vi "Plot_XY_data.vi"(0 "Channel Values":string[][](array[string]), 1 "Ordinate Strings":string[](array[string]), 2 "Swap color and symbol":i32, 3 "Error Bar Chs":i32[](array[numeric])=[11], 5 "Accept Array":bool[][](array[boolean]), 7 "Filter 1 Strings":string[](array[string]), 9 "Filter 2 Strings":string[](array[string]), 11 "Ordinate":i32[](array[numeric])=[11], 12 "Absisca":u16, 13 "Transpose":bool) -> (15 "Accept Array Out":bool[][](array[boolean]))   [LabVIEW 2010]
uses:
  Results_plotter_Global.vi
panel:
  out "Colour Array":u32[][](array[colorbox])=[[26112, 39168, 52224, 65280, 65433], [153, 13311, 26367, 52479, 65535], [16711680, 16724838, 16737894, 16737945, 16751103], [16776960, 16777062, 16777113, 16777164, 16777215], [65280, 65280, 65280, 65280, 65280], [65280, 65280, 65280, 65280, 102]]
  out "Point Choice":u8[](array[numeric])=[1, 5, 13, 2, 6, 11, 15, 14]
  in  "Index Filter2":i32
  in  "Index Filter1":i32
  in  "Index Ordinate":i32
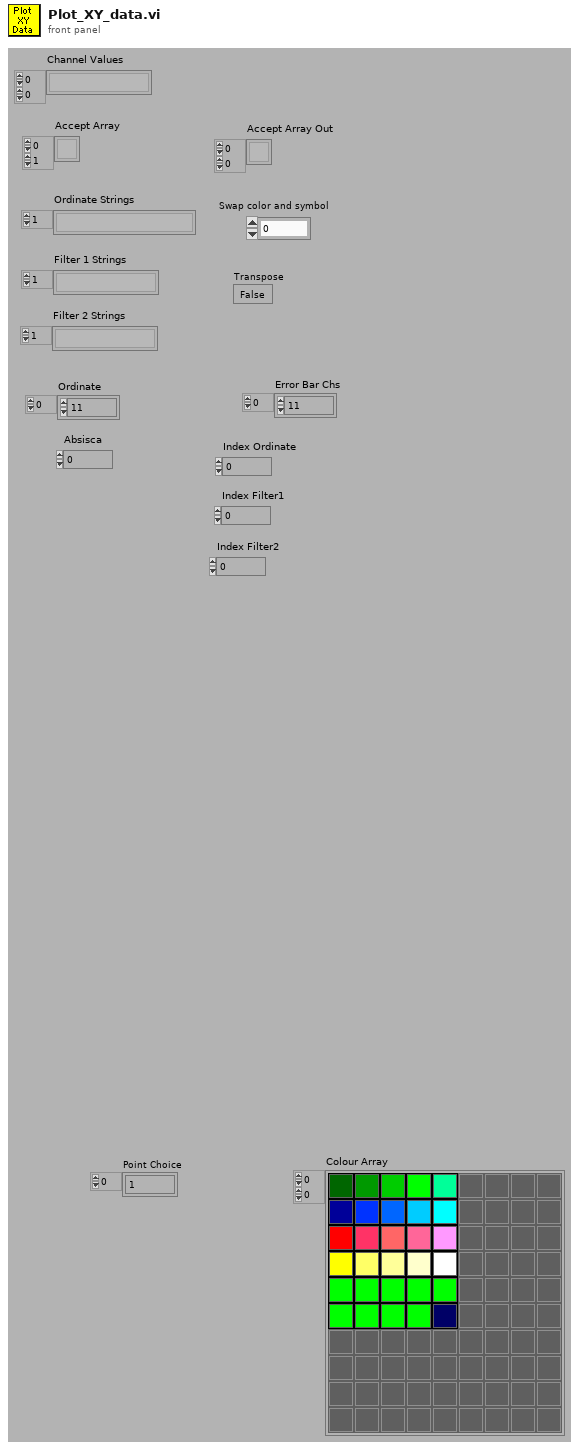
[diagram p1: front panel]
types:
  T1 = cluster{"Plot Color":u32, "Plot Interpolation":u8, "Point Style":u8, "Line Style":u8, "Fill/Pt. Color":u32, "Line Width":u8, "Bar Plot Style":u8, "Fill To":i16}
  T2 = cluster{"sorted array":dbl[], "sorted array":dbl[]}[]
  T3 = cluster{"Plot Color":u32, "Plot Interpolation":u8, "Point Style":u8, "Line Style":u8, "Fill/Pt. Color":u32, "Line Width":u8, "Bar Plot Style":u8, "Fill To":i16}[]
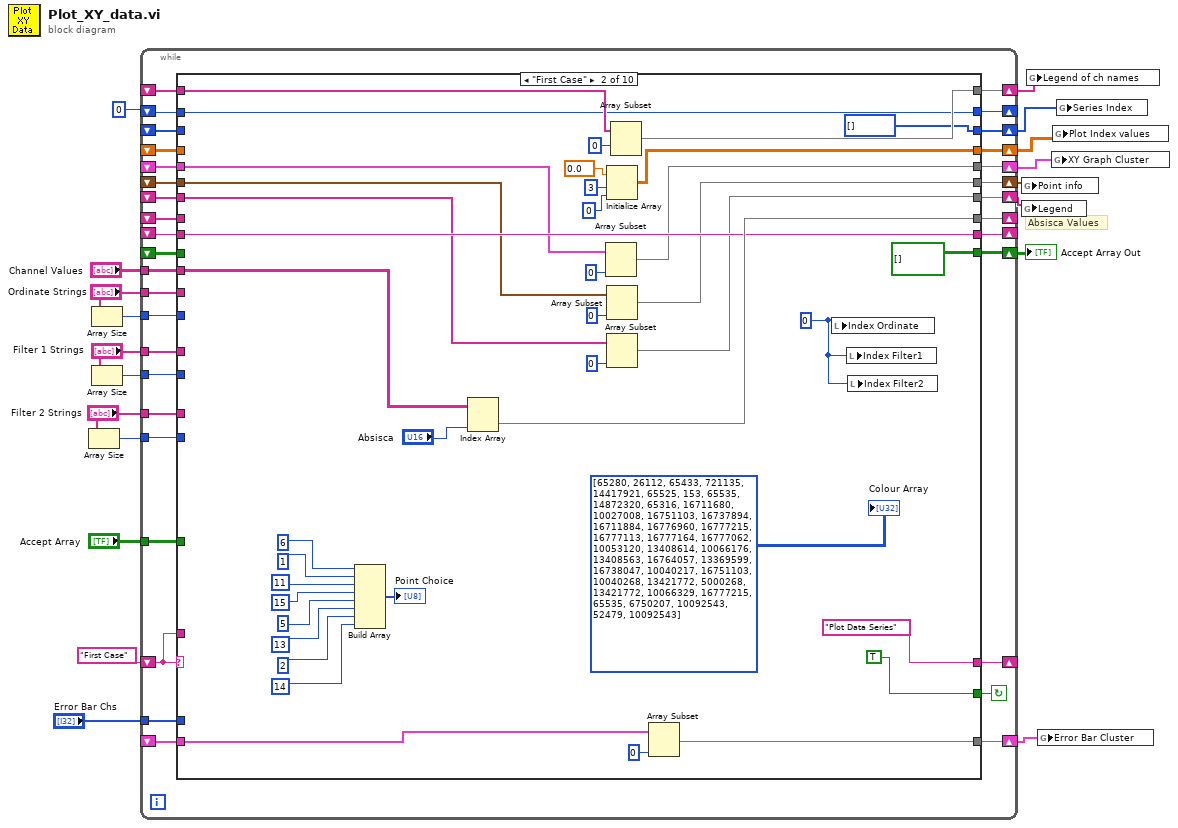
[diagram p0: block diagram]
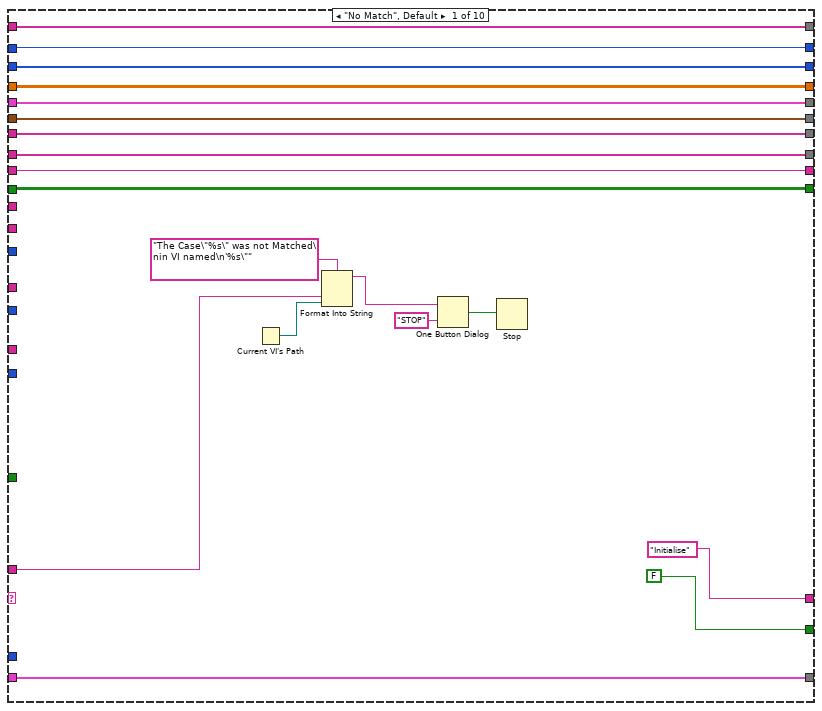
[diagram p2: hidden frame]
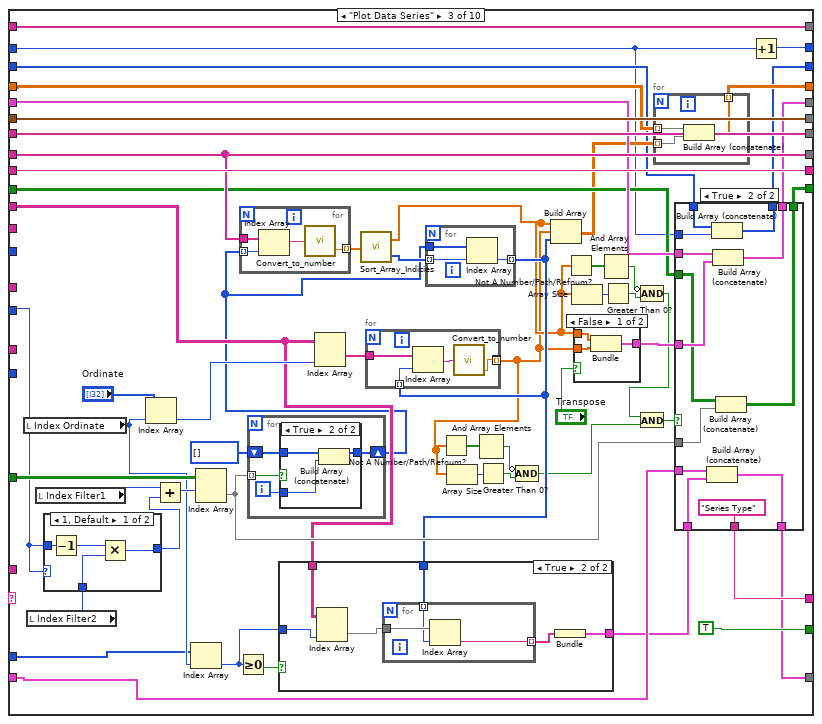
[diagram p3: hidden frame]
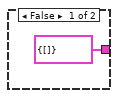
[diagram p4: hidden frame]
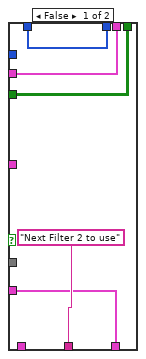
[diagram p6: hidden frame]
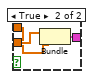
[diagram p7: hidden frame]
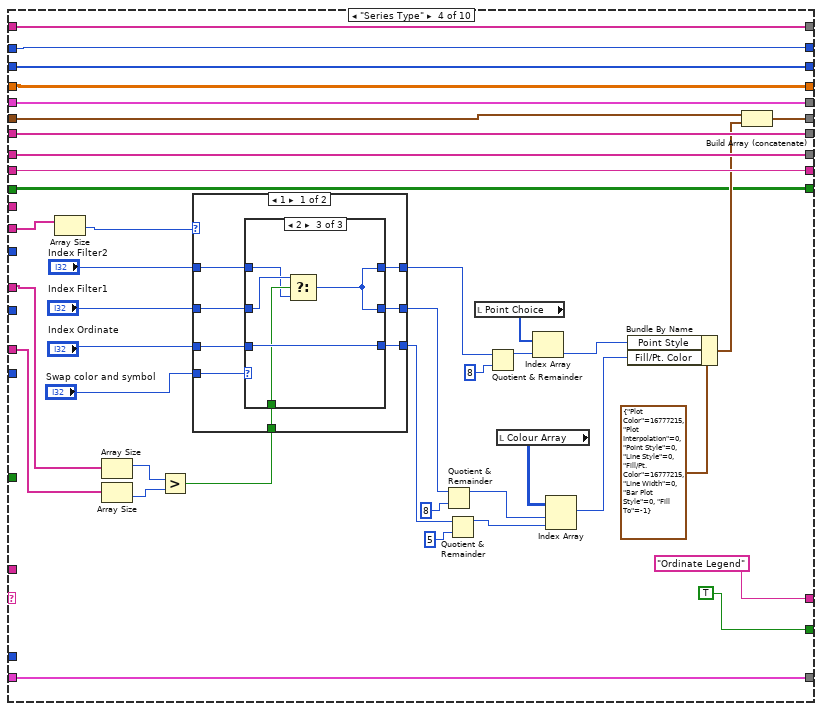
[diagram p9: hidden frame]
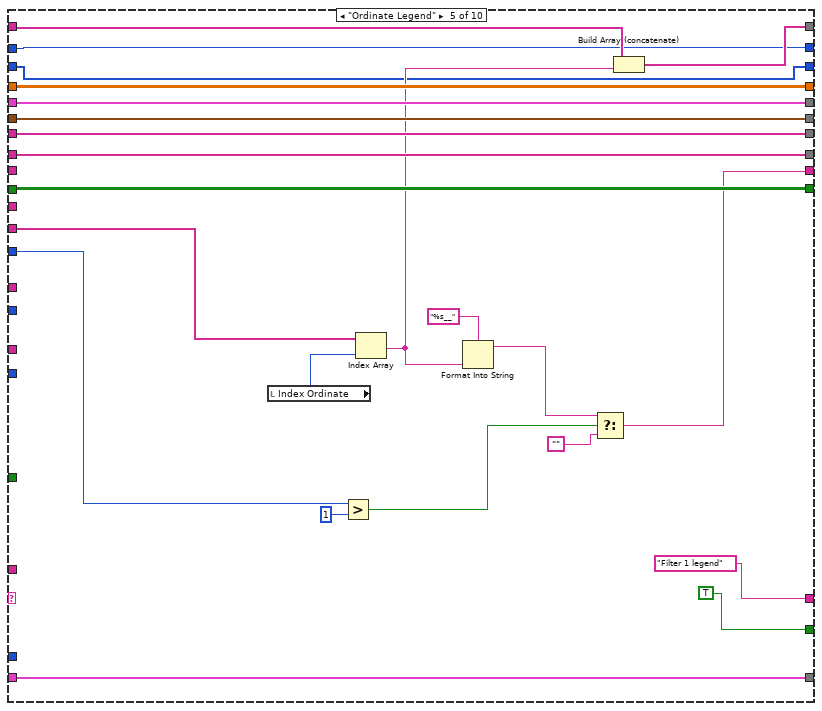
[diagram p18: hidden frame]
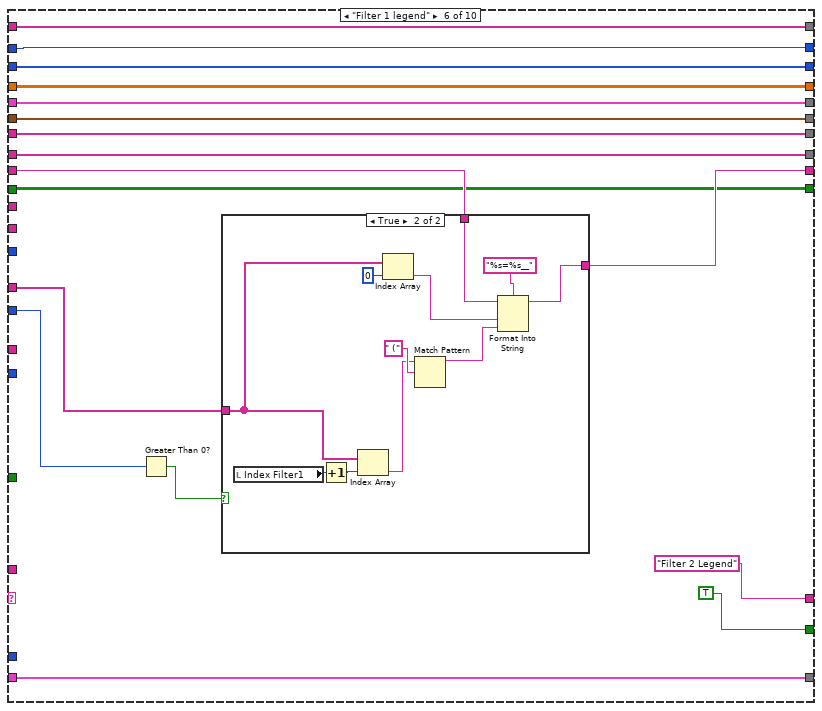
[diagram p19: hidden frame]
diagram:
  # "Absisca Values"
  n1 = Array Size(array="Filter 2 Strings") -> (size(s)=w12:i32)
  n2 = Array Size(array="Ordinate Strings") -> (size(s)=w13:i32)
  n3 = Array Size(array="Filter 1 Strings") -> (size(s)=w11:i32)
  n4 = while {
    shift-left: _ -> [w32]
    shift-right: [w31] -> w10
    tunnel: w11 -> [w33]
    tunnel: w12 -> [w34]
    tunnel: w13 -> [w35]
    tunnel: "Filter 1 Strings" -> [w36]
    tunnel: "Filter 2 Strings" -> [w37]
    tunnel: "Ordinate Strings" -> [w38]
    tunnel: "Accept Array" -> [w39]
    tunnel: "Channel Values" -> [w40]
    shift-left: _ -> [w41]
    shift-right: [w42] -> _
    shift-left: _ -> [w43]
    shift-right: [w44] -> _
    shift-left: _ -> [w46]
    shift-right: [w45] -> w7
    shift-left: _ -> [w48]
    shift-right: [w47] -> w8
    shift-left: _ -> [w50]
    shift-right: [w49] -> w6
    shift-left: "First Case" -> [w51]
    shift-right: [w52] -> _
    shift-right: [w29] -> w9
    shift-left: _ -> [w30]
    shift-right: [w28] -> w5
    shift-left: _ -> [w27]
    tunnel: "Error Bar Chs" -> [w26]
    shift-right: [w24] -> w3
    shift-left: _ -> [w25]
    shift-right: [w22] -> _
    shift-left: 0 -> [w23]
    shift-right: [w20] -> w1
    shift-left: _ -> [w21]
    stop <- w53 continue-if-true
    n5 = case shown="\"First Case\"" w51 {
      tunnel: [FALSE TRUE TRUE TRUE TRUE TRUE TRUE TRUE TRUE w450] -> w53
      tunnel: ["Initialise" "Plot Data Series" w151 "Ordinate Legend" "Filter 1 legend" "Filter 2 Legend" "Next Filter 2 to use" w402 w426 w451] -> w52
      tunnel: w51 -> [w67 _ _ _ _ _ _ _ _ _]
      tunnel: w50 -> [w64 w95 w153 w266 w333 w350 w380 w412 w436 w461]
      tunnel: [w64 w94 w152 w266 w333 w350 w380 w412 w436 w461] -> w49
      tunnel: w48 -> [w63 w90 w166 w256 w330 w347 w378 w411 w435 w460]
      tunnel: [w63 w89 w166 w254 w330 w347 w378 w411 w435 w460] -> w47
      tunnel: w46 -> [w62 w88 w165 w265 w332 w349 w372 w410 w434 w459]
      tunnel: [w62 w87 w165 w265 w332 w349 w373 w410 w434 w459] -> w45
      tunnel: [w61 w107 w161 w264 w331 w348 w379 w409 w433 w458] -> w44
      tunnel: w43 -> [w61 _ w161 w264 w331 w348 w379 w409 w433 w458]
      tunnel: [w60 w96 w164 w263 w319 w346 w371 w408 w432 w457] -> w42
      tunnel: w41 -> [w60 w96 w164 w263 _ w343 w371 w408 w432 w457]
      tunnel: w40 -> [_ w108 w136 _ _ _ _ _ _ _]
      tunnel: w39 -> [_ _ w160 _ _ _ _ _ _ _]
      tunnel: w38 -> [_ _ _ w242 w327 _ _ _ _ _]
      tunnel: w37 -> [_ _ _ w239 _ _ w376 _ _ _]
      tunnel: w36 -> [_ _ _ w240 _ w344 _ _ _ _]
      tunnel: w35 -> [_ _ _ _ w329 _ _ _ _ w448]
      tunnel: w34 -> [_ _ _ _ _ _ w375 w398 _ _]
      tunnel: w33 -> [_ _ w144 _ _ w342 _ _ w422 _]
      tunnel: w32 -> [w59 _ w149 w252 w326 w341 w370 w401 w425 w449]
      tunnel: [w59 bool[][] [] w147 w252 w326 w341 w370 w401 w425 w449] -> w31
      tunnel: w30 -> [w58 _ w141 w251 w325 w340 w369 w400 w424 w447]
      tunnel: [w58 w84 w142 w251 w325 w340 w369 w400 w424 w447] -> w29
      tunnel: w27 -> [w57 w80 w140 w232 w316 w339 w368 w399 w423 w446]
      tunnel: [w57 w75 w140 w232 w317 w339 w368 w399 w423 w446] -> w28
      tunnel: w26 -> [_ _ w138 _ _ _ _ _ _ _]
      tunnel: w25 -> [w56 w77 w134 w231 w315 w338 w367 w397 w421 w445]
      tunnel: [w56 w76 w132 w231 w315 w338 w367 w397 w421 w445] -> w24
      tunnel: w23 -> [w55 w74 w112 w230 w314 w337 w366 w396 w420 w444]
      tunnel: [w55 w74 w115 w230 w314 w337 w366 w396 w420 w444] -> w22
      tunnel: w21 -> [w54 _ w114 w229 w313 w336 w365 w395 w419 w443]
      tunnel: [w54 i32[] [] w113 w229 w313 w336 w365 w395 w419 w443] -> w20
      frame "No Match", Default {
        n6 = Current VI's Path() -> (path=w66:path)
        n7 = Format Into String(format string="The Case\"%s\" was not Matched\nin VI named\n'%s\"" ("Format String"), w67, w66) -> (resulting string=w70:string)  [unwired: 2 in, 1 out]
        n8 = One Button Dialog(message=w70, button name ("OK")="STOP") -> (true=w68:bool)
        n9 = Stop(stop? (T)=w68) -> ()
      }
      frame "First Case" {
        w106 = 0
        n10 = Build Array(u8 6 ("Write Attribute"), u8 1 ("Write Attribute"), u8 11 ("Write Attribute"), u8 15 ("Write Attribute"), u8 5 ("Write Attribute"), u8 13 ("Write Attribute"), u8 2 ("Write Attribute"), u8 14 ("Write Attribute")) -> (→"Point Choice":u8[])
        n11 = Index Array(array=w108, index (col)="Absisca") -> (element=w107:string[])  [unwired: 1 in]
        n12 = Array Subset(array=w95, length=0 ("Array Length")) -> (w94:T2)  [unwired: 1 in]
        n13 = Initialize Array(0.0 ("element"), 3 ("dimension size"), 0 ("dimension size")) -> (w84:dbl[][])
        n14 = Array Subset(array=w90, length=0 ("Array Length")) -> (w89:T3)  [unwired: 1 in]
        n15 = Array Subset(array=w88, length=0 ("Array Length")) -> (w87:string[])  [unwired: 1 in]
        n16 = Array Subset(array=w80, length=0) -> (w75:string[])  [unwired: 1 in]
        n17 = Array Subset(array=w77, length=0 ("Array Length")) -> (w76:cluster{string[]}[])  [unwired: 1 in]
        n18 = local write "Index Ordinate"(w106) -> ()
        n19 = local write "Index Filter1"(w106) -> ()
        n20 = local write "Index Filter2"(w106) -> ()
        "Colour Array" <- u32[][] [[65280, 26112, 65433, 721135, 14417921], [65525, 153, 65535, 14872320, 65316], [16711680, 10027008, 16751103, 16737894, 16711884], [16776960, 16777215, 16777113, 16777164, 16777062], [10053120, 13408614, 10066176, 13408563, 16764057], [13369599, 16738047, 10040217, 16751103, 10040268], [13421772, 5000268, 13421772, 10066329, 16777215], [65535, 6750207, 10092543, 52479, 10092543]] ("Output Array 2")
      }
      frame "Plot Data Series" {
        n21 = local read "Index Ordinate"() -> (w139:i32)
        n22 = local read "Index Filter2"() -> (w146:i32)
        n23 = local read "Index Filter1"() -> (w159:i32)
        n24 = case shown="1, Default" w144 {
          tunnel: w146 -> [w187 w188]
          tunnel: w144 -> [w186 _]
          tunnel: [w185 w188] -> w145
          frame 1, Default {
            n25 = Decrement(x=w186) -> (x-1=w184:i32)
            n26 = Multiply(x=w184, y=w187) -> (x*y=w185:i32)
          }
          frame 0 {
          }
        }
        n27 = Index Array(array="Ordinate", index=w139) -> (element=w156:i32)
        n28 = Add(x=w159, y=w145) -> (x+y=w158:i32)
        n29 = Index Array(array=w138, index=w139) -> (element=w135:i32)
        n30 = Index Array(array=w160, index (row)=w158) -> (element=w148:bool[])  [unwired: 1 in]
        n31 = Greater Or Equal To 0?(x=w135) -> (x >= 0?=w137:bool)
        n32 = for {
          shift-right: [w222] -> w129
          shift-left: i32[] [] -> [w223]
          tunnel: w148 -> [w221] mode=indexing
          i -> [w224]
          n33 = case shown="True" w221 {
            tunnel: w224 -> [_ w228]
            tunnel: w223 -> [w225 w227]
            tunnel: [w225 w226] -> w222
            frame False {
            }
            frame True {
              n34 = Build Array (concatenate)(w227, w228) -> (w226:i32[])
            }
          }
        }
        n35 = for {
          tunnel: w161 -> [w210]
          tunnel: [w208] -> w131 mode=indexing
          tunnel: w129 -> [w209] mode=indexing
          n36 = Index Array(array=w210, index=w209) -> (element=w207:string)
          n37 = call "Convert_to_number.vi"("string"=w207) -> ("Number"=w208:dbl)  [unwired: 1 out]
        }
        n38 = Index Array(array=w136, index (col)=w156) -> (element=w162:string[])  [unwired: 1 in]
        n39 = call "Sort_Array_Indicies.vi"("unsorted array"=w131) -> ("sorted array"=w127:dbl[], "Sort Index"=w130:i32[])
        n40 = for {
          tunnel: w130 -> [w170] mode=indexing
          tunnel: w129 -> [w169]
          tunnel: [w168] -> w128 mode=indexing
          n41 = Index Array(array=w169, index=w170) -> (element=w168:i32)
        }
        n42 = case shown="True" w137 {
          tunnel: w136 -> [_ w177]
          tunnel: w135 -> [_ w176]
          tunnel: w128 -> [_ w174]
          tunnel: [cluster{string[]} {[]} w173] -> w133
          frame False {
          }
          frame True {
            n43 = Index Array(array=w177, index (col)=w176) -> (element=w175:string[])  [unwired: 1 in]
            n44 = for {
              tunnel: w175 -> [w180]
              tunnel: w174 -> [w179] mode=indexing
              tunnel: [w178] -> w172 mode=indexing
              n45 = Index Array(array=w180, index=w179) -> (element=w178:string)
            }
            n46 = Bundle(w172) -> (w173:cluster{string[]})  [unwired: 1 in]
          }
        }
        n47 = for {
          tunnel: w128 -> [w220] mode=indexing
          tunnel: w162 -> [w219]
          tunnel: [w217] -> _ mode=indexing
          tunnel: [w217] -> w119 mode=indexing
          n48 = Index Array(array=w219, index=w220) -> (element=w218:string)
          n49 = call "Convert_to_number.vi"("string"=w218) -> ("Number"=w217:dbl)  [unwired: 1 out]
        }
        n50 = Not A Number/Path/Refnum?(number/path/refnum=w119) -> (NaN/Path/Refnum?=w122:bool[])
        n51 = Array Size(array=w119) -> (size(s)=w123:i32)
        n52 = And Array Elements(Boolean array=w122) -> (logical AND=w120:bool)
        n53 = Greater Than 0?(x=w123) -> (x > 0?=w121:bool)
        n54 = Compound Arithmetic op=AND(invert w120, w121) -> (w116:bool)
        n55 = Build Array(w127, w119, w128) -> (w143:dbl[][])
        n56 = Not A Number/Path/Refnum?(number/path/refnum=w127) -> (NaN/Path/Refnum?=w126:bool[])
        n57 = Array Size(array=w127) -> (size(s)=w155:i32)
        n58 = case shown="False" "Transpose" {
          tunnel: w127 -> [w213 w214]
          tunnel: [w212 w216] -> w154
          tunnel: w119 -> [w211 w215]
          frame False {
            n59 = Bundle("sorted array"=w213, w211) -> (w212:cluster{"sorted array":dbl[], dbl[]})  [unwired: 1 out]
          }
          frame True {
            n60 = Bundle(w215, "sorted array"=w214) -> (w216:cluster{dbl[], "sorted array":dbl[]})  [unwired: 1 out]
          }
        }
        n61 = And Array Elements(Boolean array=w126) -> (logical AND=w124:bool)
        n62 = Greater Than 0?(x=w155) -> (x > 0?=w125:bool)
        n63 = Compound Arithmetic op=AND(invert w124, w125) -> (w117:bool)
        n64 = And(x=w117, y=w116) -> (x .and. y?=w118:bool)
        n65 = for {
          tunnel: w141 -> [w181] mode=indexing
          tunnel: w143 -> [w183] mode=indexing
          tunnel: [w182] -> w142 mode=indexing
          n66 = Build Array (concatenate)(w181, w183) -> (w182:dbl[])
        }
        n67 = case shown="True" w118 {
          tunnel: w154 -> [_ w206]
          tunnel: w153 -> [w192 w205]
          tunnel: [w192 w197] -> w152
          tunnel: ["Next Filter 2 to use" "Series Type"] -> w151
          tunnel: w149 -> [w191 w203]
          tunnel: w148 -> [_ w202]
          tunnel: [w191 w201] -> w147
          tunnel: w134 -> [w190 w200]
          tunnel: w133 -> [_ w199]
          tunnel: [w190 w198] -> w132
          tunnel: w114 -> [w189 w196]
          tunnel: [w189 w195] -> w113
          tunnel: w112 -> [_ w194]
          frame False {
          }
          frame True {
            n68 = Build Array (concatenate)(w200, w199) -> (w198:cluster{string[]}[])
            n69 = Build Array (concatenate)(w196, w194) -> (w195:i32[])
            n70 = Build Array (concatenate)(w205, w206) -> (w197:T2)
            n71 = Build Array (concatenate)(w203, w202) -> (w201:bool[][])
          }
        }
        n72 = Increment(x=w112) -> (x+1=w115:i32)
      }
      frame "Series Type" {
        n73 = Array Size(array=w242) -> (size(s)=w241:i32)
        n74 = Array Size(array=w240) -> (size(s)=w238:i32)
        n75 = Array Size(array=w239) -> (size(s)=w237:i32)
        n76 = Greater?(x=w238, y=w237) -> (0:w236:bool)
        n77 = case shown="1" w241 {
          tunnel: [w276 w294] -> w234
          tunnel: "Index Filter2" -> [w275 w293]
          tunnel: [w274 w292] -> w247
          tunnel: "Index Filter1" -> [w273 w291]
          tunnel: "Index Ordinate" -> [w272 w290]
          tunnel: [w271 w289] -> w244
          tunnel: "Swap color and symbol" -> [w270 w288]
          tunnel: w236 -> [w269 _]
          frame 1 {
            n78 = case shown="2" w270 {
              tunnel: [w279 w281 w283] -> w276
              tunnel: w275 -> [w279 w280 w284]
              tunnel: [w278 w280 w283] -> w274
              tunnel: w273 -> [w278 w281 w285]
              tunnel: w272 -> [w277 w282 w287]
              tunnel: [w277 w282 w287] -> w271
              tunnel: w269 -> [_ _ w286]
              frame 0, Default {
              }
              frame 1 {
              }
              frame 2 {
                n79 = Select(t=w285, s=w286, f=w284) -> (s? t:f=w283:i32)
              }
            }
          }
          frame 2, Default {
            n80 = case shown="5" w288 {
              tunnel: [w297 w299 w301 w305 w309 w312] -> w294
              tunnel: w293 -> [w297 w298 w301 w304 w307 w311]
              tunnel: [w296 w298 w303 w306 w308 w311] -> w292
              tunnel: w291 -> [w296 w299 w302 w305 w308 w310]
              tunnel: w290 -> [w295 w300 w303 w306 w309 w312]
              tunnel: [w295 w300 w302 w304 w307 w310] -> w289
              frame 0, Default {
              }
              frame 1 {
              }
              frame 2 {
              }
              frame 3 {
              }
              frame 4 {
              }
              frame 5 {
              }
            }
          }
        }
        n81 = Quotient & Remainder(x=w247, y=8) -> (x-y*floor(x/y)=w250:i32)  [unwired: 1 out]
        n82 = Quotient & Remainder(x=w244, y=5) -> (x-y*floor(x/y)=w249:i32)  [unwired: 1 out]
        n83 = local read "Point Choice"() -> (w262:u8[])
        n84 = Quotient & Remainder(x=w234, y=8) -> (x-y*floor(x/y)=w233:i32)  [unwired: 1 out]
        n85 = local read "Colour Array"() -> (w259:u32[][])
        n86 = Index Array(array=w262, index=w233) -> (element=w258:u8)
        n87 = Index Array(array=w259, index (row)=w250, index (col)=w249) -> (element=w257:u32)
        n88 = Bundle By Name(cluster=T1 {"Plot Color"=16777215, "Plot Interpolation"=0, "Point Style"=0, "Line Style"=0, "Fill/Pt. Color"=16777215, "Line Width"=0, "Bar Plot Style"=0, "Fill To"=-1} ("Read Attribute"), "Point Style"=w258, "Fill/Pt. Color"=w257) -> (w255:T1)
        n89 = Build Array (concatenate)(w256, w255) -> (w254:T3)
      }
      frame "Ordinate Legend" {
        n90 = local read "Index Ordinate"() -> (w323:i32)
        n91 = Greater?(x=w329, y=1) -> (0:w322:bool)
        n92 = Index Array(array=w327, index=w323) -> (element=w318:string)
        n93 = Format Into String(format string="%s__" ("Format String"), w318) -> (resulting string=w321:string)  [unwired: 2 in, 1 out]
        n94 = Select(t=w321, s=w322, f="") -> (s? t:f=w319:string)
        n95 = Build Array (concatenate)(w316, w318) -> (w317:string[])
      }
      frame "Filter 1 legend" {
        n96 = Greater Than 0?(x=w342) -> (x > 0?=w345:bool)
        n97 = case shown="True" w345 {
          tunnel: [w353 w356] -> w346
          tunnel: w344 -> [_ w355]
          tunnel: w343 -> [w353 w360]
          frame False {
          }
          frame True {
            n98 = local read "Index Filter1"() -> (w362:i32)
            n99 = Increment(x=w362) -> (x+1=w354:i32)
            n100 = Index Array(array=w355, index=w354) -> (element=w361:string)
            n101 = Index Array(array=w355, index=0 ("Index")) -> (element=w359:string)
            n102 = Match Pattern(string=w361, regular expression=" (") -> (before substring=w357:string)  [unwired: 4 out]
            n103 = Format Into String(format string="%s=%s__" ("Format String"), initial string=w360, w359, w357) -> (resulting string=w356:string)  [unwired: 1 in, 1 out]
          }
        }
      }
      frame "Filter 2 Legend" {
        n104 = Greater Than 0?(x=w375) -> (x > 0?=w377:bool)
        n105 = case shown="False" w377 {
          tunnel: [w383 w386] -> w374
          tunnel: w376 -> [_ w385]
          tunnel: w371 -> [w383 w390]
          frame False {
          }
          frame True {
            n106 = local read "Index Filter2"() -> (w392:i32)
            n107 = Increment(x=w392) -> (x+1=w384:i32)
            n108 = Index Array(array=w385, index=w384) -> (element=w391:string)
            n109 = Index Array(array=w385, index=0 ("Index")) -> (element=w389:string)
            n110 = Match Pattern(string=w391, regular expression=" (") -> (before substring=w387:string)  [unwired: 4 out]
            n111 = Format Into String(format string="%s=%s__" ("Format String"), initial string=w390, w389, w387) -> (resulting string=w386:string)  [unwired: 1 in, 1 out]
          }
        }
        n112 = Build Array (concatenate)(w372, w374) -> (w373:string[])
      }
      frame "Next Filter 2 to use" {
        n113 = local read "Index Filter2"() -> (w404:i32)
        n114 = Add(x=w404, y=2 ("x")) -> (x+y=w407:i32)
        n115 = Less?(x=w407, y=w398) -> (x < y?=w406:bool)
        n116 = case shown="True" w406 {
          tunnel: w404 -> [_ w418]
          tunnel: [0 w417] -> w403
          tunnel: ["Next Filter 1 to use" "Plot Data Series"] -> w402
          frame False {
          }
          frame True {
            n117 = Increment(x=w418) -> (x+1=w417:i32)
          }
        }
        n118 = local write "Index Filter2"(w403) -> ()
      }
      frame "Next Filter 1 to use" {
        n119 = local read "Index Filter1"() -> (w428:i32)
        n120 = Add(x=w428, y=2 ("x")) -> (x+y=w431:i32)
        n121 = Less?(x=w431, y=w422) -> (x < y?=w430:bool)
        n122 = case shown="False" w430 {
          tunnel: w428 -> [_ w442]
          tunnel: [0 w441] -> w427
          tunnel: ["Next Ordinate" "Plot Data Series"] -> w426
          frame False {
          }
          frame True {
            n123 = Increment(x=w442) -> (x+1=w441:i32)
          }
        }
        n124 = local write "Index Filter1"(w427) -> ()
      }
      frame "Next Ordinate" {
        n125 = local read "Index Ordinate"() -> (w453:i32)
        n126 = Add(x=w453, y=1 ("x")) -> (x+y=w456:i32)
        n127 = Less?(x=w456, y=w448) -> (x < y?=w455:bool)
        n128 = case shown="False" w455 {
          tunnel: w453 -> [_ w468]
          tunnel: [0 w467] -> w452
          tunnel: ["End" "Plot Data Series"] -> w451
          tunnel: [FALSE TRUE] -> w450
          frame False {
          }
          frame True {
            n129 = Increment(x=w468) -> (x+1=w467:i32)
          }
        }
        n130 = local write "Index Ordinate"(w452) -> ()
      }
    }
  }
  "Accept Array Out" <- w10
  n131 = global write "Results_plotter_Global.vi" "Point info"(w8) -> ()
  n132 = global write "Results_plotter_Global.vi" "Legend"(w7) -> ()
  n133 = global write "Results_plotter_Global.vi" "Legend of ch names"(w5) -> ()
  n134 = global write "Results_plotter_Global.vi" "Error Bar Cluster"(w3) -> ()
  n135 = global write "Results_plotter_Global.vi" "XY Graph Cluster"(w6) -> ()
  n136 = global write "Results_plotter_Global.vi" "Plot Index values"(w9) -> ()
  n137 = global write "Results_plotter_Global.vi" "Series Index"(w1) -> ()
